vi "PI_MoveTo.vi"(0 "System no.":i32, 2 "Target position":dbl[](array[numeric]), 5 "error in":errorcluster, 6 "Move":bool) -> (14 "System no. (dup)":i32, 16 "Position":dbl[](array[numeric]), 19 "error out":errorcluster)   [LabVIEW 2010]
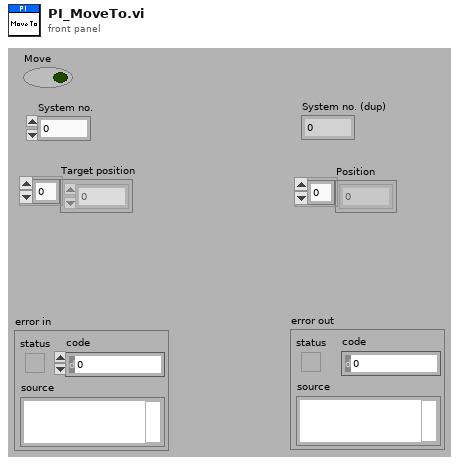
[diagram p1: front panel]
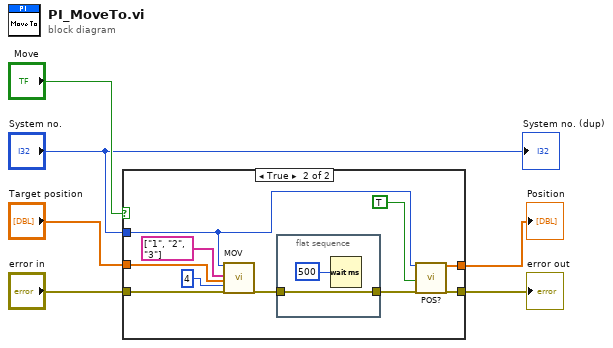
[diagram p0: block diagram]
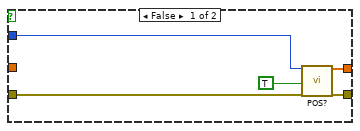
[diagram p2: hidden frame]
diagram:
  n1 = case shown="True" "Move" {
    tunnel: [w11 w16] -> w6
    tunnel: "error in" -> [w9 w21]
    tunnel: "System no." -> [w8 w15]
    tunnel: [w7 w14] -> w5
    tunnel: "Target position" -> [_ w19]
    frame False {
      n2 = call "POS?.vi"("System no."=w8, "All axes?"=TRUE, "error in"=w9) -> ("Position"=w7:dbl[], "error out"=w11:errorcluster)  [unwired: 2 in, 13 out]
    }
    frame True {
      n3 = call "MOV.vi"("System no."=w15, "Axes to move"=string[] ["1", "2", "3"], "Position values"=w19, "No.of digits"=i16 4, "error in"=w21) -> ("error out"=w13:errorcluster)  [unwired: 14 out]
      n4 = flat-sequence {
        tunnel: w13 -> [w23]
        tunnel: [w23] -> w12
        frame #0 {
          n5 = Wait (ms)(milliseconds to wait=u32 500) -> ()  [unwired: 1 out]
        }
      }
      n6 = call "POS?.vi"("System no."=w15, "All axes?"=TRUE, "error in"=w12) -> ("Position"=w14:dbl[], "error out"=w16:errorcluster)  [unwired: 2 in, 13 out]
    }
  }
  "error out" <- w6
  "Position" <- w5
  "System no. (dup)" <- "System no."
